vi "Approx Equal.vi"(2 "b":dbl, 3 "a":dbl) -> (0 "a == b?":bool)   [LabVIEW 2015]
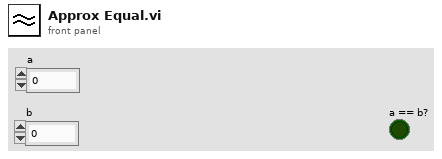
[diagram p1: front panel]
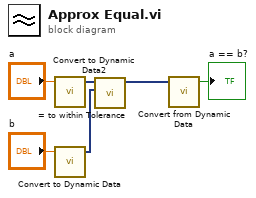
[diagram p0: block diagram]
diagram:
  n1 = call "Convert to Dynamic Data2"("Double"="a") -> ("Dynamic Data Type"=w5:dynamicdata)  [unwired: 3 in]
  n2 = call "Convert to Dynamic Data"("Double"="b") -> ("Dynamic Data Type"=w4:dynamicdata)  [unwired: 3 in]
  n3 = call "= to within Tolerance"("Operand 2"=w4, "Operand 1"=w5) -> ("Result"=w6:dynamicdata)  [unwired: 8 in, 1 out]
  n4 = call "Convert from Dynamic Data"("Dynamic Data Type"=w6) -> ("Scalar"=→"a == b?":bool)  [unwired: 3 in]
